vi "WSVCAP SHL FPGA LL I2C FIFO Manager - Transfer.vi"(7 "timeout in ms (-1)":i32, 9 "Long Word In":u64, 11 "error in (no error)":errorcluster, 13 "Operation":T1) -> (4 "Data Out":u64, 8 "Timed Out":bool, 15 "error out":errorcluster)   [LabVIEW 2017]
uses:
  Type Defs/WSVCAP SHL FIFO Operation Enum.ctl
  <vilib>/rvi/DataTransferAndStorage/Container/XNode/niFpgaContainer.xnode
  <vilib>/rvi/FIFO/Fifo_Resource/niFpgaFifoEmulationRefIn.vi
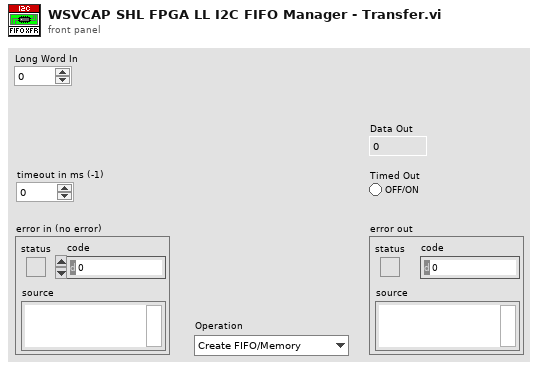
[diagram p1: front panel]
types:
  T1 = typedef "WSVCAP SHL FIFO Operation Enum.ctl" = enum16{"Create FIFO/Memory", "Get Write FIFO Status", "Get Read FIFO Status", "Put Element in Write", "Put Element in Read", "Get Element from Write", "Get Element from Read"}
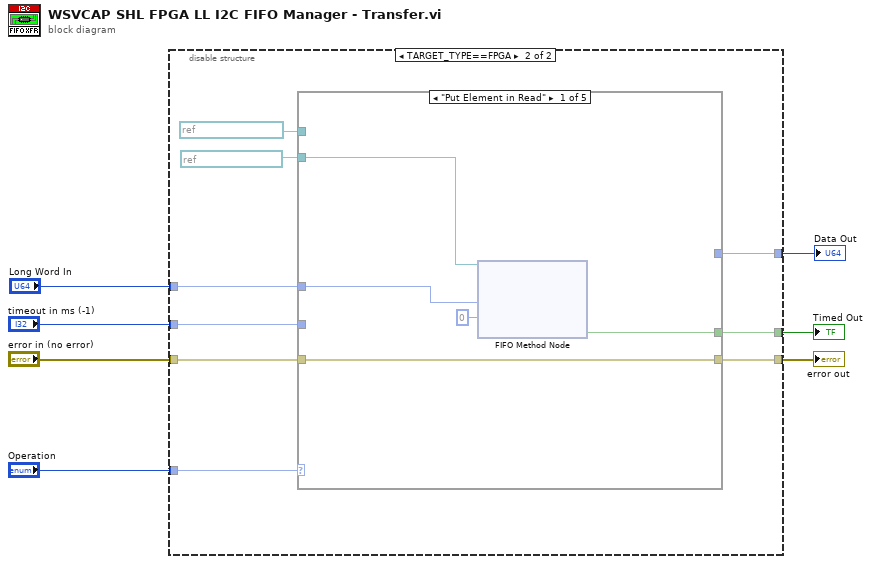
[diagram p0: block diagram]
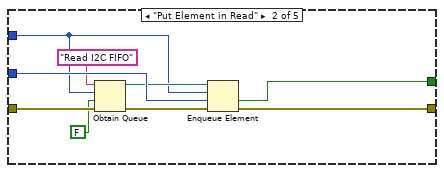
[diagram p3: hidden frame]
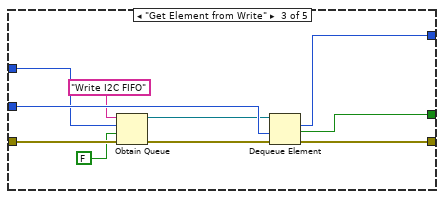
[diagram p4: hidden frame]
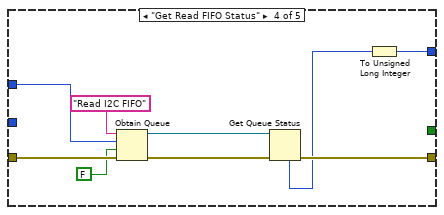
[diagram p5: hidden frame]
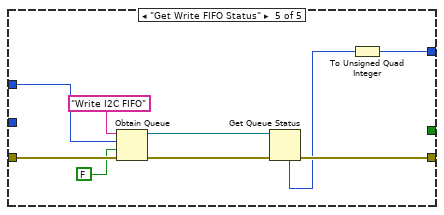
[diagram p6: hidden frame]
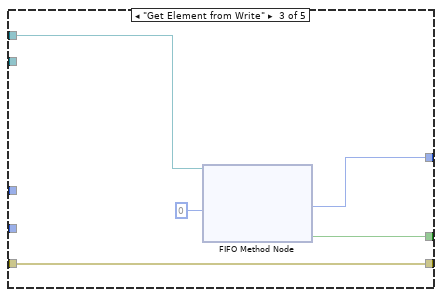
[diagram p8: hidden frame]
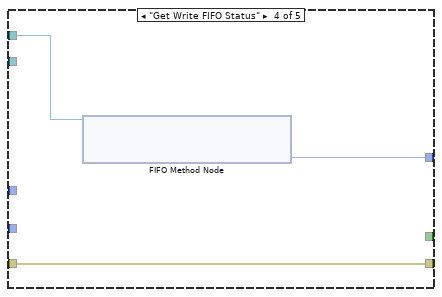
[diagram p9: hidden frame]
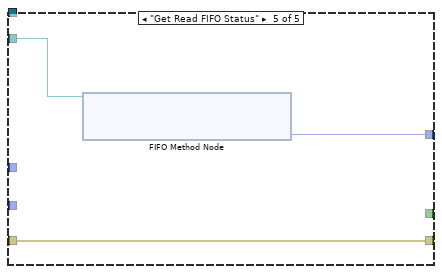
[diagram p10: hidden frame]
diagram:
  n1 = disable-structure shown="TARGET_TYPE==FPGA" {
    disable-tunnel: "Operation" -> [w14 w61]
    disable-tunnel: "error in (no error)" -> [w13 w58]
    disable-tunnel: [w12 w57] -> w5
    disable-tunnel: "timeout in ms (-1)" -> [w11 w60]
    disable-tunnel: [w10 w56] -> w3
    disable-tunnel: [w9 w59] -> w2
    disable-tunnel: "Long Word In" -> [w8 w55]
    frame condition #0 (active) {
      n2 = case shown="Default" w14 {
        tunnel: [w15 w24 w33 w43 w52] -> w12
        tunnel: w13 -> [w15 w21 w30 w42 w51]
        tunnel: w11 -> [_ w23 w34 _ _]
        tunnel: [_ _ w32 w36 w45] -> w10
        tunnel: [_ w22 w31 _ _] -> w9
        tunnel: w8 -> [_ w16 w27 w39 w48]
        frame Default {
        }
        frame "Put Element in Read" {
          n3 = Obtain Queue(name (unnamed)="Read I2C FIFO", element data type=w16, create if not found? (T)=FALSE, error in (no error)=w21) -> (queue out=w19:refnum<queue>, error out=w20:errorcluster)  [unwired: 1 in, 1 out]
          n4 = Enqueue Element(queue=w19, element=w16, timeout in ms (-1)=w23, error in (no error)=w20) -> (timed out?=w22:bool, error out=w24:errorcluster)  [unwired: 1 out]
        }
        frame "Get Element from Write" {
          n5 = Obtain Queue(name (unnamed)="Write I2C FIFO", element data type=w27, create if not found? (T)=FALSE, error in (no error)=w30) -> (queue out=w26:refnum<queue>, error out=w25:errorcluster)  [unwired: 1 in, 1 out]
          n6 = Dequeue Element(queue=w26, timeout in ms (-1)=w34, error in (no error)=w25) -> (element=w32:u64, timed out?=w31:bool, error out=w33:errorcluster)  [unwired: 1 out]
        }
        frame "Get Read FIFO Status" {
          n7 = Obtain Queue(name (unnamed)="Read I2C FIFO", element data type=w39, create if not found? (T)=FALSE, error in (no error)=w42) -> (queue out=w38:refnum<queue>, error out=w37:errorcluster)  [unwired: 1 in, 1 out]
          n8 = Get Queue Status(queue=w38, error in (no error)=w37) -> (error out=w43:errorcluster, # elements in queue=w35:i32)  [unwired: 1 in, 6 out]
          n9 = To Unsigned Long Integer(number=w35) -> (unsigned 32bit integer=w36:u32)
        }
        frame "Get Write FIFO Status" {
          n10 = Obtain Queue(name (unnamed)="Write I2C FIFO", element data type=w48, create if not found? (T)=FALSE, error in (no error)=w51) -> (queue out=w47:refnum<queue>, error out=w46:errorcluster)  [unwired: 1 in, 1 out]
          n11 = Get Queue Status(queue=w47, error in (no error)=w46) -> (error out=w52:errorcluster, # elements in queue=w44:i32)  [unwired: 1 in, 6 out]
          n12 = To Unsigned Quad Integer(1:w44) -> (0:w45:u64)
        }
      }
    }
    frame condition #1 {
      n13 = case shown="\"Put Element in Read\"" w61 {
        tunnel: w60 -> [_ _ _ _ _]
        tunnel: [w65 _ w71 _ _] -> w59
        tunnel: w58 -> [w62 w67 w68 w73 w78]
        tunnel: [w62 w67 w68 w73 w78] -> w57
        tunnel: [_ _ w69 w75 w76] -> w56
        tunnel: w55 -> [w66 _ _ _ _]
        tunnel: refnum<k21> "I2C_Read Data" ("FIFO In") -> [w63 _ _ _ w77]
        tunnel: refnum<k21> "I2C_Write Data" ("FIFO In") -> [_ _ w70 w74 _]
        frame "Put Element in Read" {
          n14 = xnode ("FIFO Method Node")("Element"=w66, "Timeout"=0, "FIFO In"=w63) -> ("Timed Out?"=w65:bool)  [unwired: 1 out]
        }
        frame Default {
        }
        frame "Get Element from Write" {
          n15 = xnode ("FIFO Method Node")("Timeout"=0, "FIFO In"=w70) -> ("Element"=w69:u64, "Timed Out?"=w71:bool)  [unwired: 1 out]
        }
        frame "Get Write FIFO Status" {
          n16 = xnode ("FIFO Method Node")("FIFO In"=w74) -> ("Number of Elements to Read"=w75:u32)  [unwired: 1 out]
        }
        frame "Get Read FIFO Status" {
          n17 = xnode ("FIFO Method Node")("FIFO In"=w77) -> ("Number of Elements to Read"=w76:u32)  [unwired: 1 out]
        }
      }
    }
  }
  "error out" <- w5
  "Data Out" <- w3
  "Timed Out" <- w2
